vi "report data.vi"() -> (1 "VW_ Medium":T1, 6 "Data":string[](array[string]))   [LabVIEW 2015]
uses:
  Galobal variable_TI.vi
panel:
  out "size(s)":i32
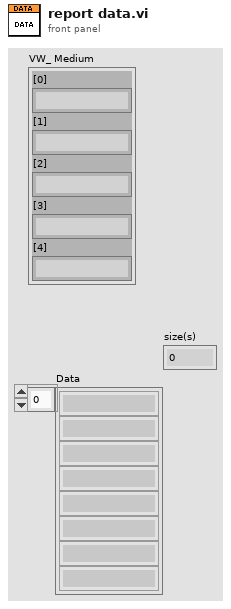
[diagram p1: front panel]
types:
  T1 = cluster{"[0]":string, "[1]":string, "[2]":string, "[3]":string, "[4]":string}
  T2 = cluster{"LVDT1Max(mm) AI0":dbl, "LVDT1Min (mm)AI0":dbl, "LVDT2Max(mm) AI1":dbl, "LVDT2Min(mm) AI1":dbl, "LVDT3Max(mm) AI2":dbl, "LVDT3Min(mm) AI2":dbl, "LVDT4Max(mm) AI3":dbl, "LVDT4Min(mm) AI3":dbl, "Model":string, "MIC Code":string}
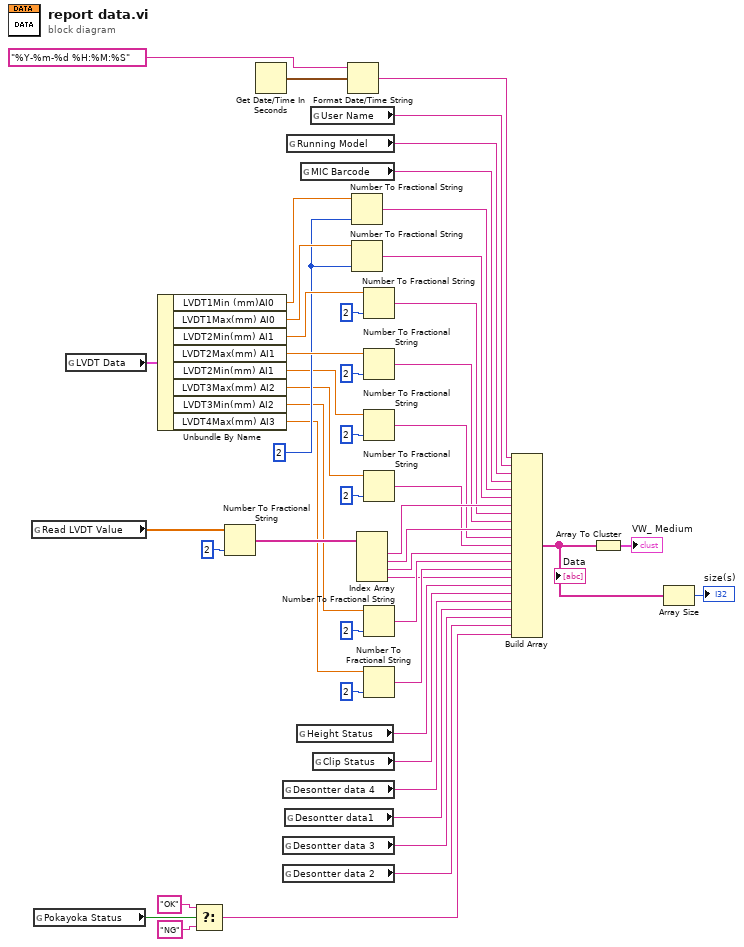
[diagram p0: block diagram]
diagram:
  w33 = i16 2 ("precision (6)")
  n1 = global read "Galobal variable_TI.vi" "Read LVDT Value"() -> (w32:dbl[])
  n2 = global read "Galobal variable_TI.vi" "Pokayoka Status"() -> (w41:bool)
  n3 = global read "Galobal variable_TI.vi" "LVDT Data"() -> (w50:T2)
  n4 = Unbundle By Name(w50) -> ("LVDT1Min (mm)AI0"=w49:dbl, "LVDT1Max(mm) AI0"=w46:dbl, "LVDT2Min(mm) AI1"=w45:dbl, "LVDT2Max(mm) AI1"=w44:dbl, "LVDT2Min(mm) AI1"=w24:dbl, "LVDT3Max(mm) AI2"=w23:dbl, "LVDT3Min(mm) AI2"=w14:dbl, "LVDT4Max(mm) AI3"=w13:dbl)
  n5 = Select(t="OK", s=w41, f="NG") -> (s? t:f=w3:string)
  n6 = Number To Fractional String(number=w32, precision (6)=i16 2) -> (F-format string=w30:string[])  [unwired: 2 in]
  n7 = Get Date/Time In Seconds() -> (seconds since 1Jan1904=w37:timestamp)
  n8 = global read "Galobal variable_TI.vi" "Desontter data 4"() -> (w7:string)
  n9 = global read "Galobal variable_TI.vi" "Desontter data 3"() -> (w5:string)
  n10 = global read "Galobal variable_TI.vi" "Desontter data 2"() -> (w4:string)
  n11 = global read "Galobal variable_TI.vi" "Desontter data1"() -> (w6:string)
  n12 = global read "Galobal variable_TI.vi" "Running Model"() -> (w39:string)
  n13 = global read "Galobal variable_TI.vi" "Height Status"() -> (w9:string)
  n14 = global read "Galobal variable_TI.vi" "MIC Barcode"() -> (w38:string)
  n15 = global read "Galobal variable_TI.vi" "User Name"() -> (w40:string)
  n16 = global read "Galobal variable_TI.vi" "Clip Status"() -> (w8:string)
  n17 = Format Date/Time String(time format string (%c)="%Y-%m-%d %H:%M:%S", seconds (now)=w37) -> (date/time string=w36:string)  [unwired: 1 in]
  n18 = Number To Fractional String(number=w49, precision (6)=w33) -> (F-format string=w29:string)  [unwired: 2 in]
  n19 = Number To Fractional String(number=w46, precision (6)=w33) -> (F-format string=w28:string)  [unwired: 2 in]
  n20 = Index Array(array=w30) -> (element #1=w27:string, element #2=w20:string, element #3=w17:string, element #4=w10:string)  [unwired: 4 in]
  n21 = Number To Fractional String(number=w45, precision (6)=i16 2) -> (F-format string=w22:string)  [unwired: 2 in]
  n22 = Number To Fractional String(number=w44, precision (6)=i16 2) -> (F-format string=w21:string)  [unwired: 2 in]
  n23 = Number To Fractional String(number=w24, precision (6)=i16 2) -> (F-format string=w19:string)  [unwired: 2 in]
  n24 = Number To Fractional String(number=w23, precision (6)=i16 2) -> (F-format string=w18:string)  [unwired: 2 in]
  n25 = Number To Fractional String(number=w14, precision (6)=i16 2) -> (F-format string=w12:string)  [unwired: 2 in]
  n26 = Number To Fractional String(number=w13, precision (6)=i16 2) -> (F-format string=w11:string)  [unwired: 2 in]
  n27 = Build Array(w36, w40, w39, w38, w29, w28, w27, w22, w21, w20, w19, w18, w17, w12, w11, w10, w9, w8, w7, w6, w5, w4, w3) -> (w2:string[])
  "Data" <- w2
  n28 = Array To Cluster(array=w2) -> (cluster=→"VW_ Medium":T1)
  n29 = Array Size(array=w2) -> (size(s)=→"size(s)":i32)
